vi "GetHelp.vi"(11 "RunTests in":refnum<class "RunVITester.lvclass">) -> (2 "Help out":string, 3 "RunTests out":refnum<class "RunVITester.lvclass">)   [LabVIEW 2027, in "RunVITester.lvclass"]
uses:
  RunVITester.lvclass
panel:
  in  "Help in":string="LabVIEWCLI -OperationName RunVITester -TestPath <path of the test case to run> -ReportPath <path of the test report>\n\n -TestPath  Path of the VI Tester test case to run. One or more TestPath must be specified.\n-ReportPath   Path of the JUnit XML file test report to generate. A temporary location will be generated if none is specified."
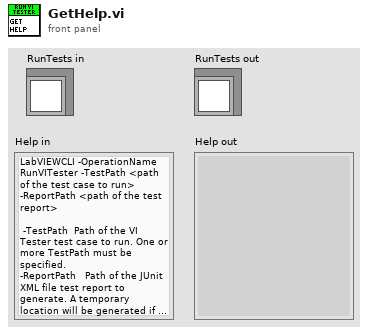
[diagram p1: front panel]
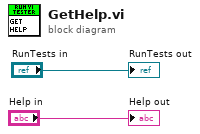
[diagram p0: block diagram]
diagram:
  "RunTests out" <- "RunTests in"
  "Help out" <- "Help in"
